vi "main_power_gauge.vi"() -> ()   [LabVIEW 2009]
uses:
  <vilib>/Utility/file.llb/Write To Spreadsheet File (DBL).vi
panel:
  out "Testmessung [mW]":dbl
  out "Vektor Position [°]":dbl[](array[numeric])
  out "Vektor Leistung [mW]":dbl[](array[numeric])
  out "Aktuelle Position [°]":dbl format="%_4g"
  out "XY-Graph":T1(graph)
  out "Aktueller Messschritt":u64
  out "Leistung [mW]":dbl format="%#_4g"
  out "Messung gestartet":bool
  out "Messende [°]":dbl
  in  "Start [°]":dbl
  in  "Messung ON/OFF":bool
  in  "Messungen/Schritt":u64=20
  out "Bühne und Powermeter initialisiert":bool
  in  "SN von Rotationsbühne":i32=83831982
  in  "Rotation stage":refnum<k7>(container) caption="Aktuelle Position [°]"
  in  "# Schritte":u64=73
  in  "Schrittweite [°]":dbl=5.0
  in  "Programm beenden":bool
  out "Powermeter":refnum<visa-resource-name>
  in  "Powermeter Anschluss":string="ASRL3::INSTR"
  # "COM2 Anschluss ist zweiter, vertikaler Anschluss von rechts (PC von hinten betrachtet)"
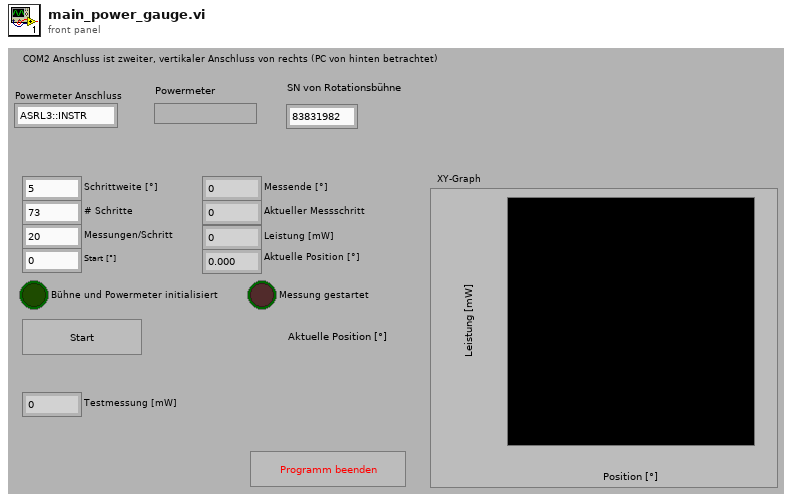
[diagram p1: front panel]
types:
  T1 = cluster{"Vektor Leistung [mW] ":dbl[], "Vektor Position [°]":dbl[]}
  T2 = cluster{"Vektor Position [°]":dbl[], "Vektor Leistung [mW] ":dbl[]}
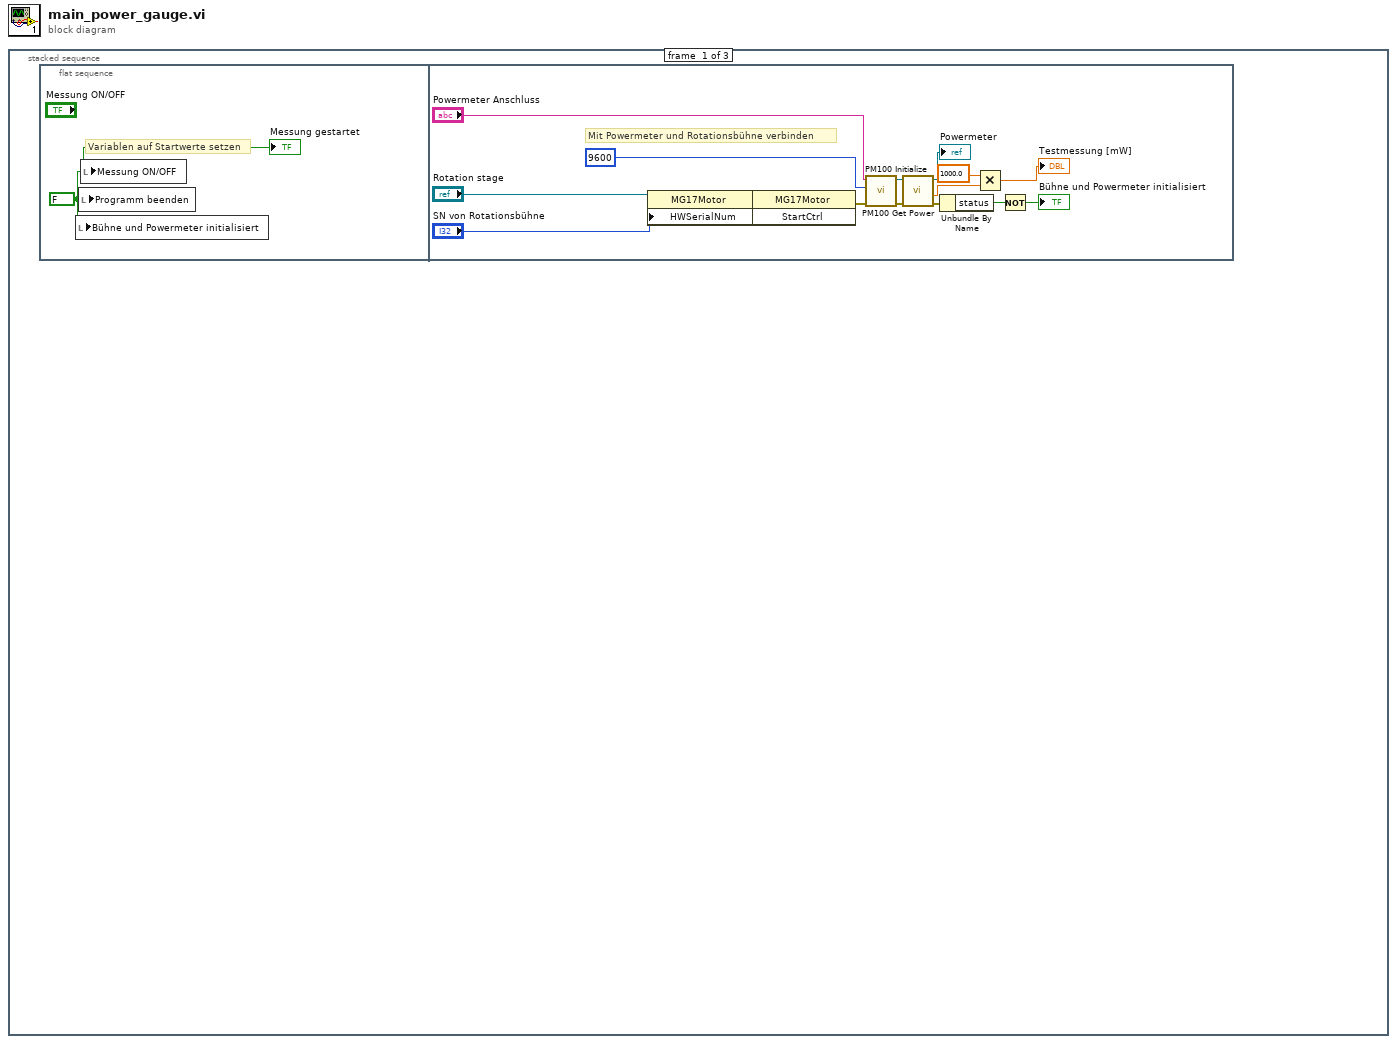
[diagram p0: block diagram]
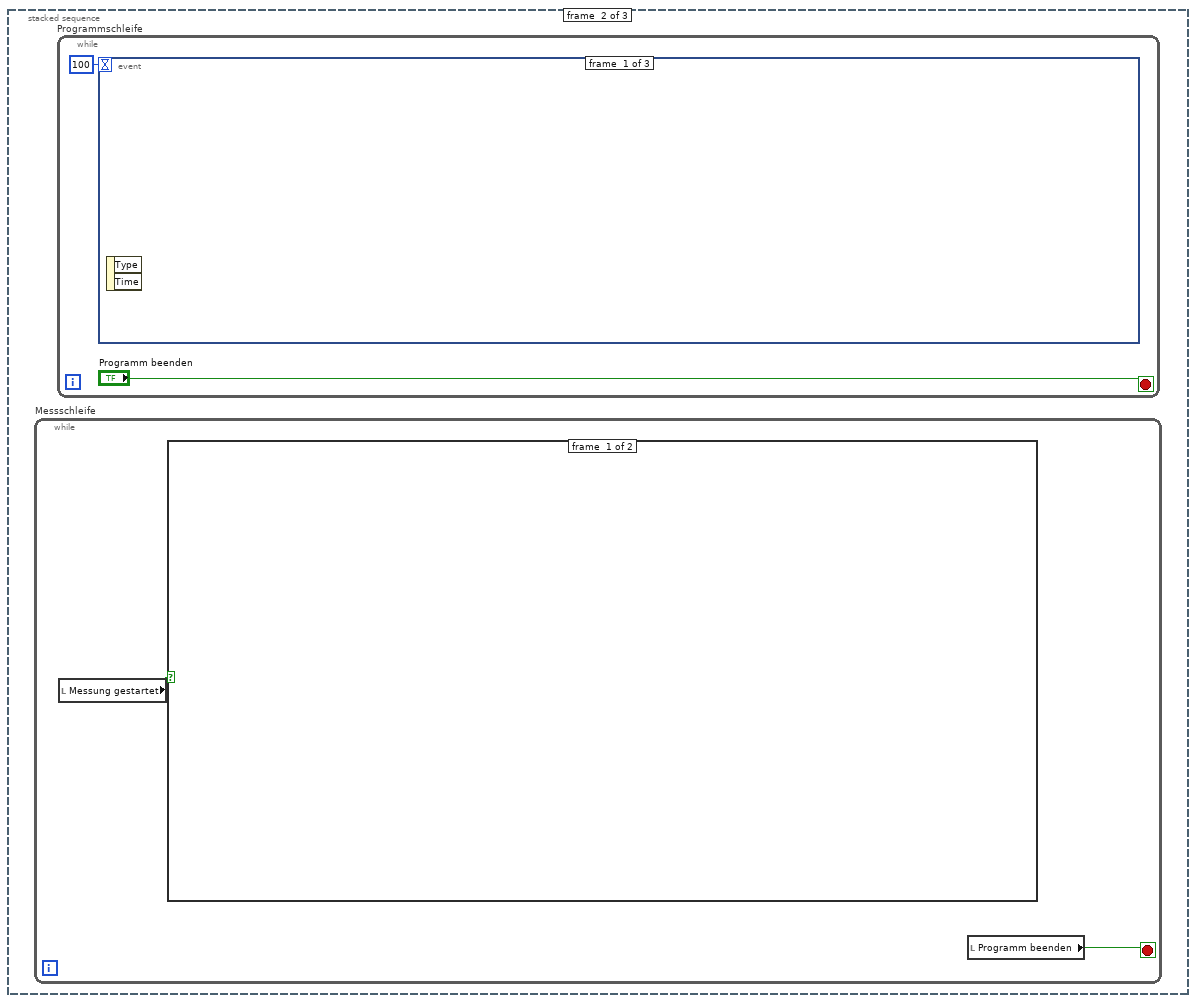
[diagram p2: hidden frame]
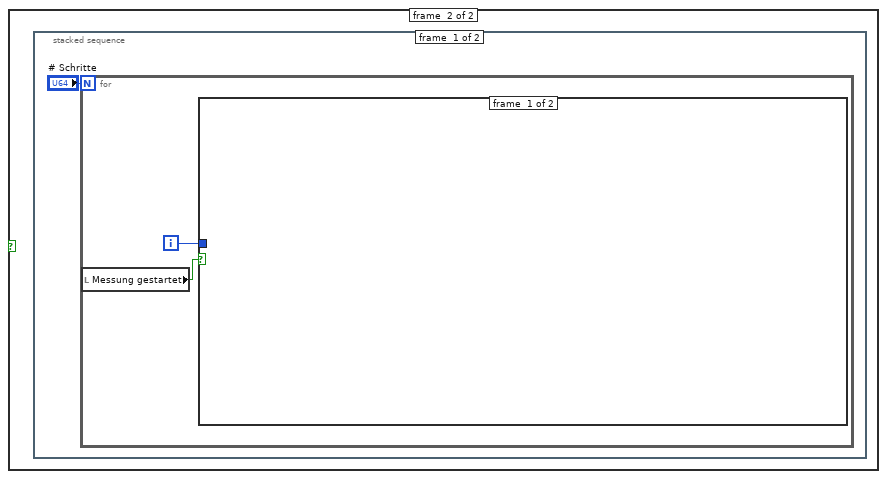
[diagram p3: hidden frame]
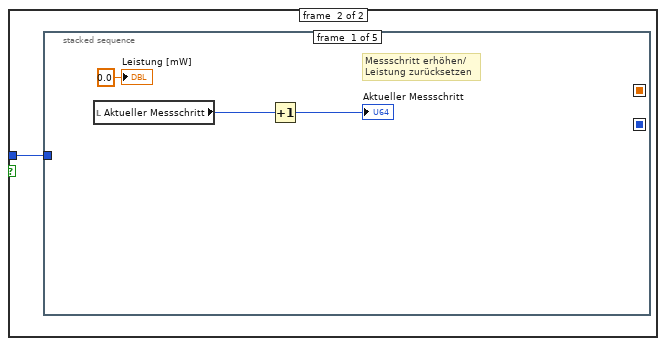
[diagram p4: hidden frame]
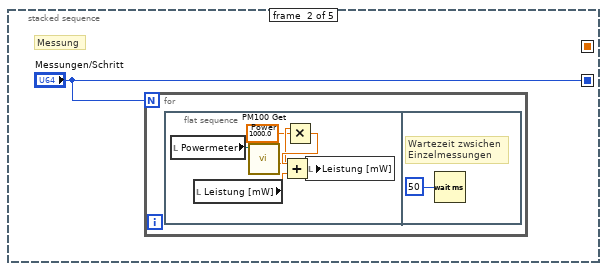
[diagram p5: hidden frame]
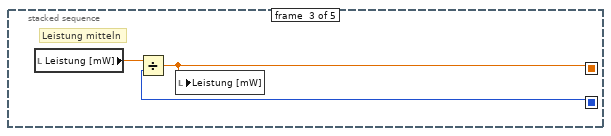
[diagram p6: hidden frame]
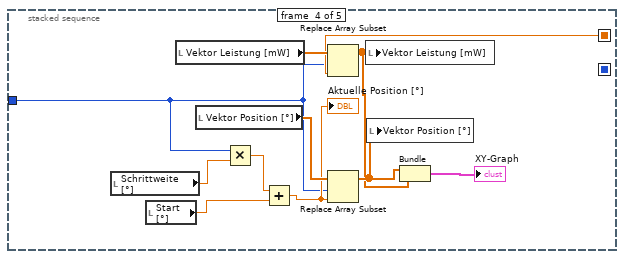
[diagram p7: hidden frame]
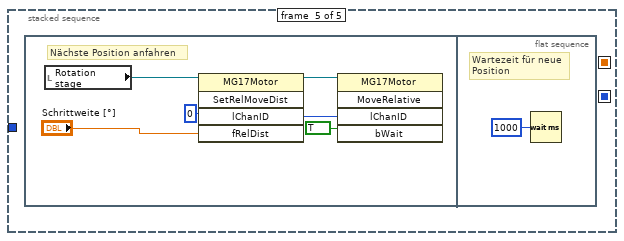
[diagram p8: hidden frame]
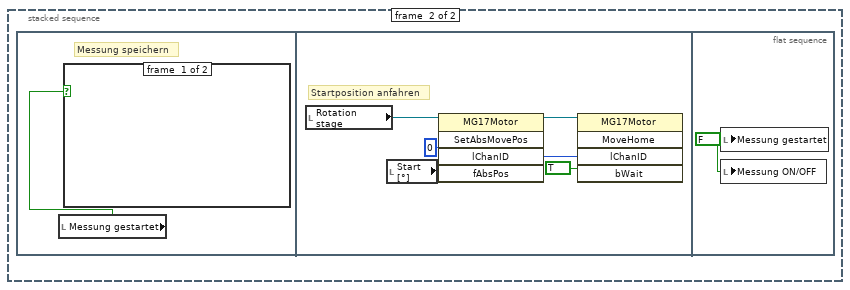
[diagram p9: hidden frame]
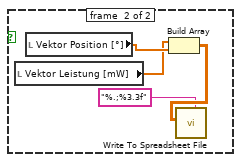
[diagram p10: hidden frame]
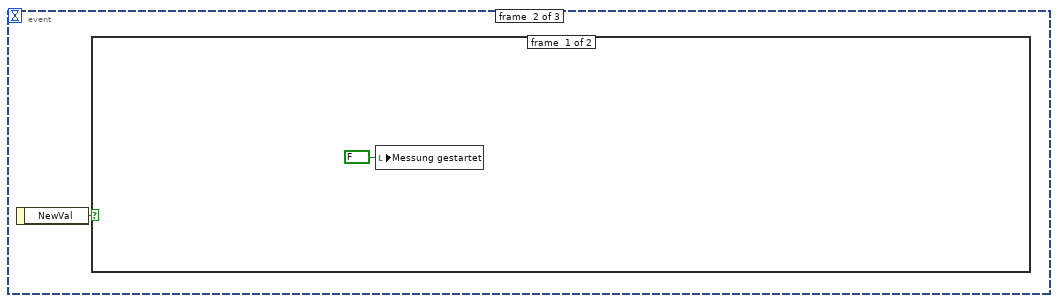
[diagram p11: hidden frame]
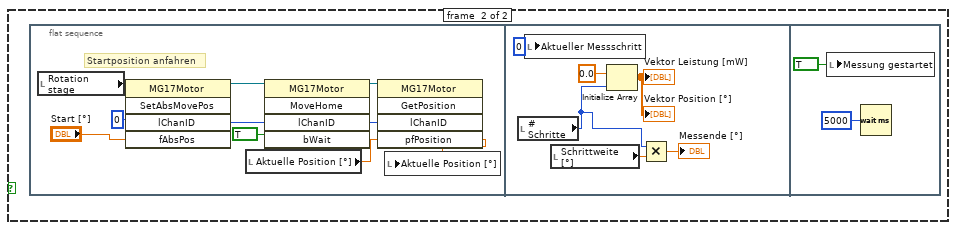
[diagram p12: hidden frame]
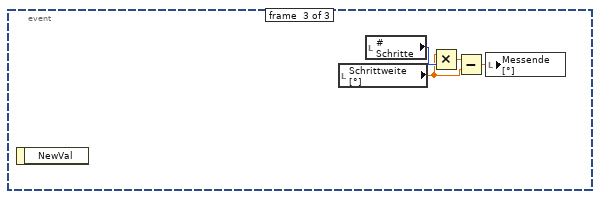
[diagram p13: hidden frame]
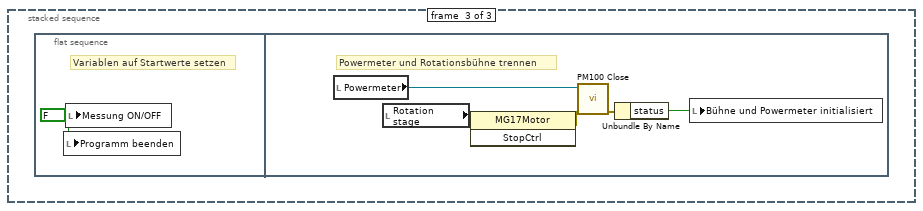
[diagram p14: hidden frame]
diagram:
  n1 = stacked-sequence {
    frame #0 {
      n2 = flat-sequence {
        frame #0 {
          w1 = FALSE ("Bühne und Powermeter initialisiert")
          # "Variablen auf Startwerte setzen"
          n3 = local write "Bühne und Powermeter initialisiert"(w1) -> ()
          n4 = local write "Programm beenden"(w1) -> ()
          n5 = local write "Messung ON/OFF"(w1) -> ()
          "Messung gestartet" <- w1
        }
        frame #1 {
          # "Mit Powermeter und Rotationsbühne verbinden"
          n6 = property class="MG17Motor"(reference="Rotation stage", "HWSerialNum"="SN von Rotationsbühne") -> (reference out=w15:refnum<k7>, error out=w14:errorcluster)  [unwired: 1 in]
          n7 = invoke class="MG17Motor" method="StartCtrl"(reference=w15, error in=w14) -> (error out=w11:errorcluster)  [unwired: 1 in, 2 out]
          n8 = call <userlib>:"PM100 Initialize.vi"("error in (no error)"=w11, "baudrate"=9600, "resource name"="Powermeter Anschluss") -> ("error out"=w7:errorcluster, "instrument handle out"=w8:refnum<visa-resource-name>)  [unwired: 6 in, 1 out]
          n9 = call <userlib>:"PM100 Get Power.vi"("error in (no error)"=w7, "instrument handle"=w8) -> ("error out"=w4:errorcluster, "power"=w5:dbl, "instrument handle out"=→"Powermeter":refnum<visa-resource-name>)  [unwired: 6 in, 1 out]
          n10 = Unbundle By Name(w4) -> ("status"=w9:bool)
          n11 = Multiply(x=1000.0, y=w5) -> (x*y=→"Testmessung [mW]":dbl)
          n12 = Not(x=w9) -> (.not. x?=→"Bühne und Powermeter initialisiert":bool)
        }
      }
    }
    frame #1 {
      n13 = while "Messschleife" {
        stop <- w18 stop-if-true
        n14 = local read "Messung gestartet"() -> (w19:bool)
        n15 = case shown="True" w19 {
          frame #0 {
          }
          frame #1 {
            n16 = stacked-sequence {
              frame #0 {
                n17 = for {
                  N: "# Schritte" -> [_]
                  i -> [w22]
                  n18 = local read "Messung gestartet"() -> (w21:bool)
                  n19 = case shown="True" w21 {
                    tunnel: w22 -> [_ w23]
                    frame #0 {
                    }
                    frame #1 {
                      n20 = stacked-sequence {
                        seq-local: [_ "Messungen/Schritt" _ _ _] -> [_ _ w36 _ _]
                        seq-local: [_ _ w35 _ _] -> [_ _ _ w46 _]
                        tunnel: w23 -> [_ _ _ w39 _]
                        frame #0 {
                          # "Messschritt erhöhen/\nLeistung zurücksetzen"
                          n21 = local read "Aktueller Messschritt"() -> (w24:u64)
                          n22 = Increment(x=w24) -> (x+1=→"Aktueller Messschritt":u64)
                          "Leistung [mW]" <- 0.0 ("Leistung [mW]")
                        }
                        frame #1 {
                          # "Messung"
                          n23 = for {
                            N: "Messungen/Schritt" -> [_]
                            n24 = flat-sequence {
                              frame #0 {
                                n25 = local read "Powermeter"() -> (w33:refnum<visa-resource-name>)
                                n26 = local read "Leistung [mW]"() -> (w32:dbl)
                                n27 = call <userlib>:"PM100 Get Power.vi"("instrument handle"=w33) -> ("power"=w29:dbl)  [unwired: 7 in, 3 out]
                                n28 = Multiply(x=w29, y=1000.0) -> (x*y=w30:dbl)
                                n29 = Add(x=w30, y=w32) -> (x+y=w31:dbl)
                                n30 = local write "Leistung [mW]"(w31) -> ()
                              }
                              frame #1 {
                                # "Wartezeit zwsichen\nEinzelmessungen"
                                n31 = Wait (ms)(milliseconds to wait=u32 50 ("Zu wartende ms")) -> ()  [unwired: 1 out]
                              }
                            }
                          }
                        }
                        frame #2 {
                          # "Leistung mitteln"
                          n32 = local read "Leistung [mW]"() -> (w37:dbl)
                          n33 = Divide(x=w37, y=w36) -> (x/y=w35:dbl)
                          n34 = local write "Leistung [mW]"(w35) -> ()
                        }
                        frame #3 {
                          n35 = local read "Schrittweite [°]"() -> (w40:dbl)
                          n36 = local read "Start [°]"() -> (w42:dbl)
                          n37 = local read "Vektor Leistung [mW]"() -> (w48:dbl[])
                          n38 = local read "Vektor Position [°]"() -> (w47:dbl[])
                          n39 = Multiply(x=w39, y=w40) -> (x*y=w38:dbl)
                          n40 = Add(x=w38, y=w42) -> (x+y=w41:dbl)
                          "Aktuelle Position [°]" <- w41
                          n41 = Replace Array Subset(array=w48, new element=w46, index=w39) -> (w43:dbl[])
                          n42 = Replace Array Subset(array=w47, new element=w41, index=w39) -> (w44:dbl[])
                          n43 = local write "Vektor Leistung [mW]"(w43) -> ()
                          n44 = local write "Vektor Position [°]"(w44) -> ()
                          n45 = Bundle("Vektor Position [°]"=w44, "Vektor Leistung [mW]"=w43) -> (→"XY-Graph":T2)  [unwired: 1 in]
                        }
                        frame #4 {
                          n46 = flat-sequence {
                            frame #0 {
                              # "Nächste Position anfahren"
                              n47 = local read "Rotation stage"() -> (w50:refnum<k7>)
                              n48 = invoke class="MG17Motor" method="SetRelMoveDist"(reference=w50, "lChanID"=0, "fRelDist"="Schrittweite [°]") -> (reference out=w51:refnum<k7>, "lChanID"=w53:i32)  [unwired: 2 in, 3 out]
                              n49 = invoke class="MG17Motor" method="MoveRelative"(reference=w51, "lChanID"=w53, "bWait"=TRUE) -> ()  [unwired: 2 in, 5 out]
                            }
                            frame #1 {
                              # "Wartezeit für neue\nPosition"
                              n50 = Wait (ms)(milliseconds to wait=u32 1000 ("Zu wartende ms")) -> ()  [unwired: 1 out]
                            }
                          }
                        }
                      }
                    }
                  }
                }
              }
              frame #1 {
                n51 = flat-sequence {
                  frame #0 {
                    # "Messung speichern"
                    n52 = local read "Messung gestartet"() -> (w56:bool)
                    n53 = case shown="True" w56 {
                      frame #0 {
                      }
                      frame #1 {
                        n54 = local read "Vektor Leistung [mW]"() -> (w59:dbl[])
                        n55 = local read "Vektor Position [°]"() -> (w60:dbl[])
                        n56 = Build Array(w59, w60) -> (w58:dbl[][])
                        n57 = call-poly <vilib>:"Write To Spreadsheet File.vi"("format (%.3f)"="%.;%3.3f", "2D data"=w58) -> ()  [unwired: 6 in, 1 out]
                      }
                    }
                  }
                  frame #1 {
                    # "Startposition anfahren"
                    n58 = local read "Rotation stage"() -> (w66:refnum<k7>)
                    n59 = local read "Start [°]"() -> (w61:dbl)
                    n60 = invoke class="MG17Motor" method="SetAbsMovePos"(reference=w66, "lChanID"=0, "fAbsPos"=w61) -> (reference out=w63:refnum<k7>, "lChanID"=w65:i32)  [unwired: 2 in, 3 out]
                    n61 = invoke class="MG17Motor" method="MoveHome"(reference=w63, "lChanID"=w65, "bWait"=TRUE) -> ()  [unwired: 2 in, 5 out]
                  }
                  frame #2 {
                    w67 = FALSE ("Messung gestartet")
                    n62 = local write "Messung gestartet"(w67) -> ()
                    n63 = local write "Messung ON/OFF"(w67) -> ()
                  }
                }
              }
            }
          }
        }
        n64 = local read "Programm beenden"() -> (w18:bool)
      }
      n65 = while "Programmschleife" {
        stop <- "Programm beenden" stop-if-true
        n66 = event shown="[1] \"Messung ON/OFF\": Wertänderung" {
          selector: _ -> [_ _ _]
          dyn-events: _ -> [_ _ _]
          timeout: 100 -> [_ _ _]
          event #0 {
            n67 = event-data() -> ()  [unwired: 1 in, 2 out]
          }
          event #1 {
            n68 = event-data() -> ("NewVal"=w70:bool)  [unwired: 1 in]
            n69 = case shown="True" w70 {
              frame #0 {
                n70 = local write "Messung gestartet"(FALSE ("Messung gestartet")) -> ()
              }
              frame #1 {
                n71 = flat-sequence {
                  frame #0 {
                    # "Startposition anfahren"
                    n72 = local read "Rotation stage"() -> (w76:refnum<k7>)
                    n73 = invoke class="MG17Motor" method="SetAbsMovePos"(reference=w76, "lChanID"=0, "fAbsPos"="Start [°]") -> (reference out=w80:refnum<k7>, "lChanID"=w77:i32)  [unwired: 2 in, 3 out]
                    n74 = local read "Aktuelle Position [°]"() -> (w73:dbl)
                    n75 = invoke class="MG17Motor" method="MoveHome"(reference=w80, "lChanID"=w77, "bWait"=TRUE) -> (reference out=w75:refnum<k7>, "lChanID"=w74:i32)  [unwired: 2 in, 3 out]
                    n76 = invoke class="MG17Motor" method="GetPosition"(reference=w75, "lChanID"=w74, "pfPosition"=w73) -> ("pfPosition"=w72:sgl)  [unwired: 2 in, 4 out]
                    n77 = local write "Aktuelle Position [°]"(w72) -> ()
                  }
                  frame #1 {
                    n78 = local read "# Schritte"() -> (w82:u64)
                    n79 = local write "Aktueller Messschritt"(u64 0 ("Aktueller Messschritt")) -> ()
                    n80 = local read "Schrittweite [°]"() -> (w87:dbl)
                    n81 = Initialize Array(0.0 ("Element"), w82) -> (→"Vektor Leistung [mW]" →"Vektor Position [°]":dbl[])
                    n82 = Multiply(x=w82, y=w87) -> (x*y=→"Messende [°]":dbl)
                  }
                  frame #2 {
                    n83 = local write "Messung gestartet"(TRUE ("Messung gestartet")) -> ()
                    n84 = Wait (ms)(milliseconds to wait=u32 5000 ("Zu wartende ms")) -> ()  [unwired: 1 out]
                  }
                }
              }
            }
          }
          event #2 {
            n85 = event-data() -> ()  [unwired: 1 in, 1 out]
            n86 = local read "Schrittweite [°]"() -> (w91:dbl)
            n87 = local read "# Schritte"() -> (w93:u64)
            n88 = Multiply(x=w91, y=w93) -> (x*y=w92:dbl)
            n89 = Subtract(x=w92, y=w91) -> (x-y=w90:dbl)
            n90 = local write "Messende [°]"(w90) -> ()
          }
        }
      }
    }
    frame #2 {
      n91 = flat-sequence {
        frame #0 {
          w94 = FALSE ("Bühne und Powermeter initialisiert")
          # "Variablen auf Startwerte setzen"
          n92 = local write "Programm beenden"(w94) -> ()
          n93 = local write "Messung ON/OFF"(w94) -> ()
        }
        frame #1 {
          # "Powermeter und Rotationsbühne trennen"
          n94 = local read "Powermeter"() -> (w98:refnum<visa-resource-name>)
          n95 = local read "Rotation stage"() -> (w99:refnum<k7>)
          n96 = invoke class="MG17Motor" method="StopCtrl"(reference=w99) -> (error out=w97:errorcluster)  [unwired: 2 in, 2 out]
          n97 = call <userlib>:"PM100 Close.vi"("error in (no error)"=w97, "instrument handle"=w98) -> ("error out"=w96:errorcluster)  [unwired: 8 in, 1 out]
          n98 = Unbundle By Name(w96) -> ("status"=w95:bool)
          n99 = local write "Bühne und Powermeter initialisiert"(w95) -> ()
        }
      }
    }
  }
